vi "Configure Digital Voltmeter.vi"(7 "Auto Range (F: Disable)":bool, 8 "error in (no error)":errorcluster, 9 "Source Channel (0: Channel 1)":i32(ring) items=["Channel 1", "Channel 2", "Channel 3", "Channel 4"], 10 "Digital Voltmeter Type (4: OFF)":i32(ring)=4 items=["ACRMS", "ACDCRMS", "DC", "Frequency", "Off"], 11 "VISA resource name":refnum<visa-resource-name>) -> (0 "error out":errorcluster, 3 "VISA resource name out":refnum<visa-resource-name>)   [LabVIEW 2017, in "Scope.lvlib" / "Tektronix DPO MSO 2000 4000 Series.lvlib"]
doc: "Configures the Digital Voltmeter.\n\n<B>Notes:</B>\n(1) This VI is available for MDO3000 Series only.\n\n(2) Requires the MDO3AFG option to be installed."
uses:
  Tektronix DPO MSO 2000 4000 Series.lvlib
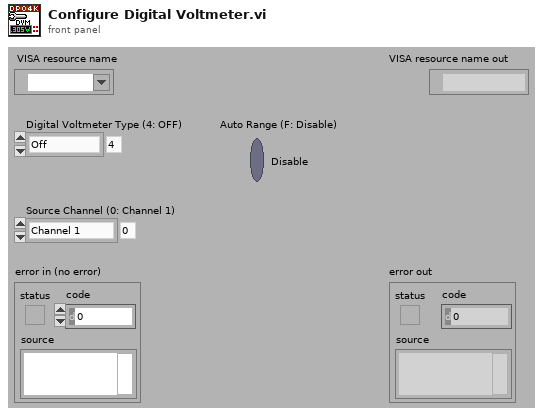
[diagram p1: front panel]
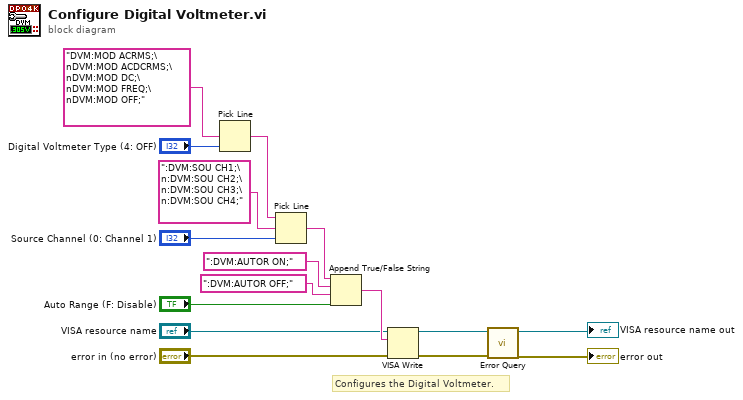
[diagram p0: block diagram]
diagram:
  # "Configures the Digital Voltmeter."
  n1 = Pick Line(multi-line string="DVM:MOD ACRMS;\nDVM:MOD ACDCRMS;\nDVM:MOD DC;\nDVM:MOD FREQ;\nDVM:MOD OFF;", line index="Digital Voltmeter Type (4: OFF)") -> (output string=w12:string)  [unwired: 1 in]
  n2 = Pick Line(string ("")=w12, multi-line string=":DVM:SOU CH1;\n:DVM:SOU CH2;\n:DVM:SOU CH3;\n:DVM:SOU CH4;", line index="Source Channel (0: Channel 1)") -> (output string=w11:string)
  n3 = Append True/False String(1:"Auto Range (F: Disable)", 2:":DVM:AUTOR OFF;", 3:":DVM:AUTOR ON;", 4:w11) -> (0:w7:string)
  n4 = VISA Write(VISA resource name="VISA resource name", write buffer=w7, error in (no error)="error in (no error)") -> (VISA resource name out=w5:refnum<visa-resource-name>, error out=w4:errorcluster)  [unwired: 1 out]
  n5 = call "Error Query.vi"("error in (no error)"=w4, "VISA resource name"=w5) -> ("error out"=→"error out":errorcluster, "VISA resource name out"=→"VISA resource name out":refnum<visa-resource-name>)  [unwired: 6 in, 2 out]
